vi "CC Obervation Generate Dither Step.vi"(8 "error in (no error)":errorcluster, 11 "Dither Options":T1) -> (0 "error out":errorcluster, 2 "Name":string, 3 "Step":T4={"Action"=enum."Acquire Images", "Data"=variant})   [LabVIEW 2024]
uses:
  typedefs/CC Script Step.ctl
  typedefs/CC enum Script Action.ctl
  typedefs/CC cluster Observation Dither Options.ctl
  typedefs/CC enum Dither Selection.ctl
  typedefs/CC cluster RA and DEC.ctl
  typedefs/CC Dithering.ctl
  typedefs/CC cluster Offset Dithering.ctl
  typedefs/CC Dithering Offsets.ctl
  typedefs/CC cluster Random Dithering.ctl
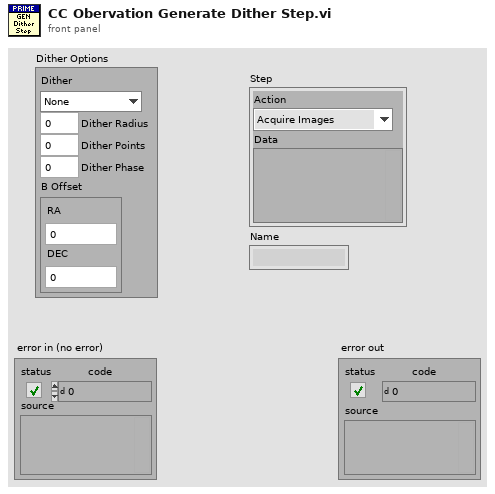
[diagram p1: front panel]
types:
  T1 = typedef "CC cluster Observation Dither Options.ctl" = cluster{"Dither":T2, "Dither Radius":dbl, "Dither Points":i32, "Dither Phase":dbl, "B Offset":T3}
  T2 = typedef "CC enum Dither Selection.ctl" = enum16{"None", "Circle", "Random", "ABBA", "OnOff"}
  T3 = typedef "CC cluster RA and DEC.ctl" = cluster{"RA":dbl, "DEC":dbl}
  T4 = typedef "CC Script Step.ctl" = cluster{"Action":T5, "Data":variant}
  T5 = typedef "CC enum Script Action.ctl" = enum16{"Noop", "Define Object", "Define Exposure", "Define Dithering", "Acquire Images", "Set Filter Wheel", "Telescope Home", "Telescope Move", "Telescope RA DEC", "Focus Move Relative", "Focus Move Absolute", "Focus Set Home", "Macro", "Pause", "Ask User", "Define Random Dither", "CmdLine", "Outlet"}
  T6 = typedef "CC Dithering.ctl" = cluster{"Name":string, "Dithering Offsets":T7}
  T7 = typedef "CC cluster Offset Dithering.ctl" = cluster{"Offsets":T8[]}
  T8 = typedef "CC Dithering Offsets.ctl" = cluster{"DEC":dbl, "RA":dbl}
  T9 = typedef "CC cluster Random Dithering.ctl" = cluster{"Count":i32, "Radius":dbl, "Name":string}
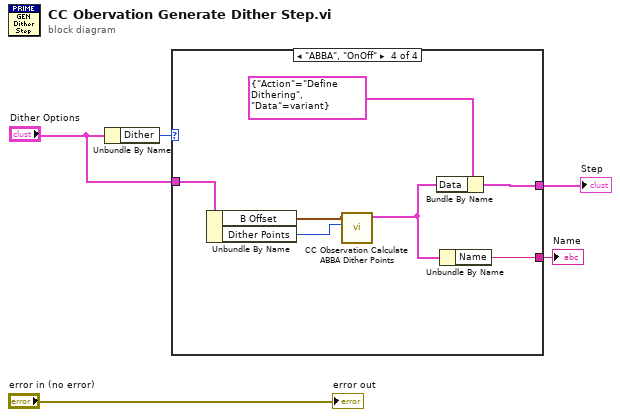
[diagram p0: block diagram]
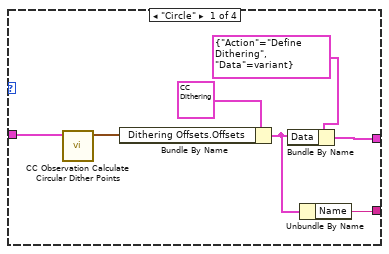
[diagram p2: hidden frame]
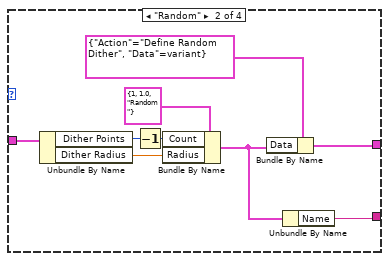
[diagram p3: hidden frame]
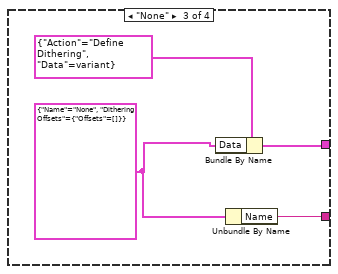
[diagram p4: hidden frame]
diagram:
  n1 = Unbundle By Name("Dither Options") -> ("Dither"=w4:T2)
  n2 = case shown="\"ABBA\", \"OnOff\"" w4 {
    tunnel: "Dither Options" -> [w12 w20 _ w29]
    tunnel: [w8 w16 w24 w31] -> w2
    tunnel: [w6 w14 w23 w30] -> w1
    frame "Circle" {
      n3 = call "CC Observation Calculate Circular Dither Points.vi"("Dither Options"=w12) -> ("Points"=w10:T8[])  [unwired: 9 in, 1 out]
      n4 = Bundle By Name(cluster=T6 {"Name"="Circle", "Dithering Offsets"={"Offsets"=[{"DEC"=-1.0, "RA"=-1.0}, {"DEC"=-1.0, "RA"=1.0}, {"DEC"=1.0, "RA"=1.0}, {"DEC"=1.0, "RA"=-1.0}]}} ("Dithering Offsets"), "Dithering Offsets.Offsets"=w10) -> (w7:T6)
      n5 = Bundle By Name(cluster=T4 {"Action"=enum."Define Dithering", "Data"=variant}, "Data"=w7) -> (w8:T4)
      n6 = Unbundle By Name(w7) -> ("Name"=w6:string)
    }
    frame "Random" {
      n7 = Unbundle By Name(w20) -> ("Dither Points"=w18:i32, "Dither Radius"=w17:dbl)
      n8 = Decrement(x=w18) -> (x-1=w13:i32)
      n9 = Bundle By Name(cluster=T9 {"Count"=1, "Radius"=1.0, "Name"="Random"} ("Random Dither"), "Count"=w13, "Radius"=w17) -> (w15:T9)
      n10 = Bundle By Name(cluster=T4 {"Action"=enum."Define Random Dither", "Data"=variant}, "Data"=w15) -> (w16:T4)
      n11 = Unbundle By Name(w15) -> ("Name"=w14:string)
    }
    frame "None" {
      w22 = T6 {"Name"="None", "Dithering Offsets"={"Offsets"=[]}} ("Dithering Offsets")
      n12 = Bundle By Name(cluster=T4 {"Action"=enum."Define Dithering", "Data"=variant}, "Data"=w22) -> (w24:T4)
      n13 = Unbundle By Name(w22) -> ("Name"=w23:string)
    }
    frame "ABBA", "OnOff" {
      n14 = Unbundle By Name(w29) -> ("B Offset"=w28:T3, "Dither Points"=w26:i32)
      n15 = call "CC Observation Calculate ABBA Dither Points.vi"("# Points"=w26, "B Offset"=w28) -> ("Dither"=w27:T6)  [unwired: 8 in, 1 out]
      n16 = Bundle By Name(cluster=T4 {"Action"=enum."Define Dithering", "Data"=variant}, "Data"=w27) -> (w31:T4)
      n17 = Unbundle By Name(w27) -> ("Name"=w30:string)
    }
  }
  "Step" <- w2
  "Name" <- w1
  "error out" <- "error in (no error)"
